vi "商品生成.vi"(11 "天数":i32 min=0 max=31) -> (2 "物品存在索引":i32[](array[numeric]), 3 "市面商品":string[][](array[string]))   [LabVIEW 2011]
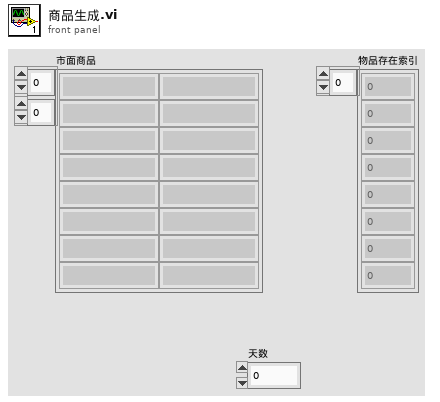
[diagram p1: front panel]
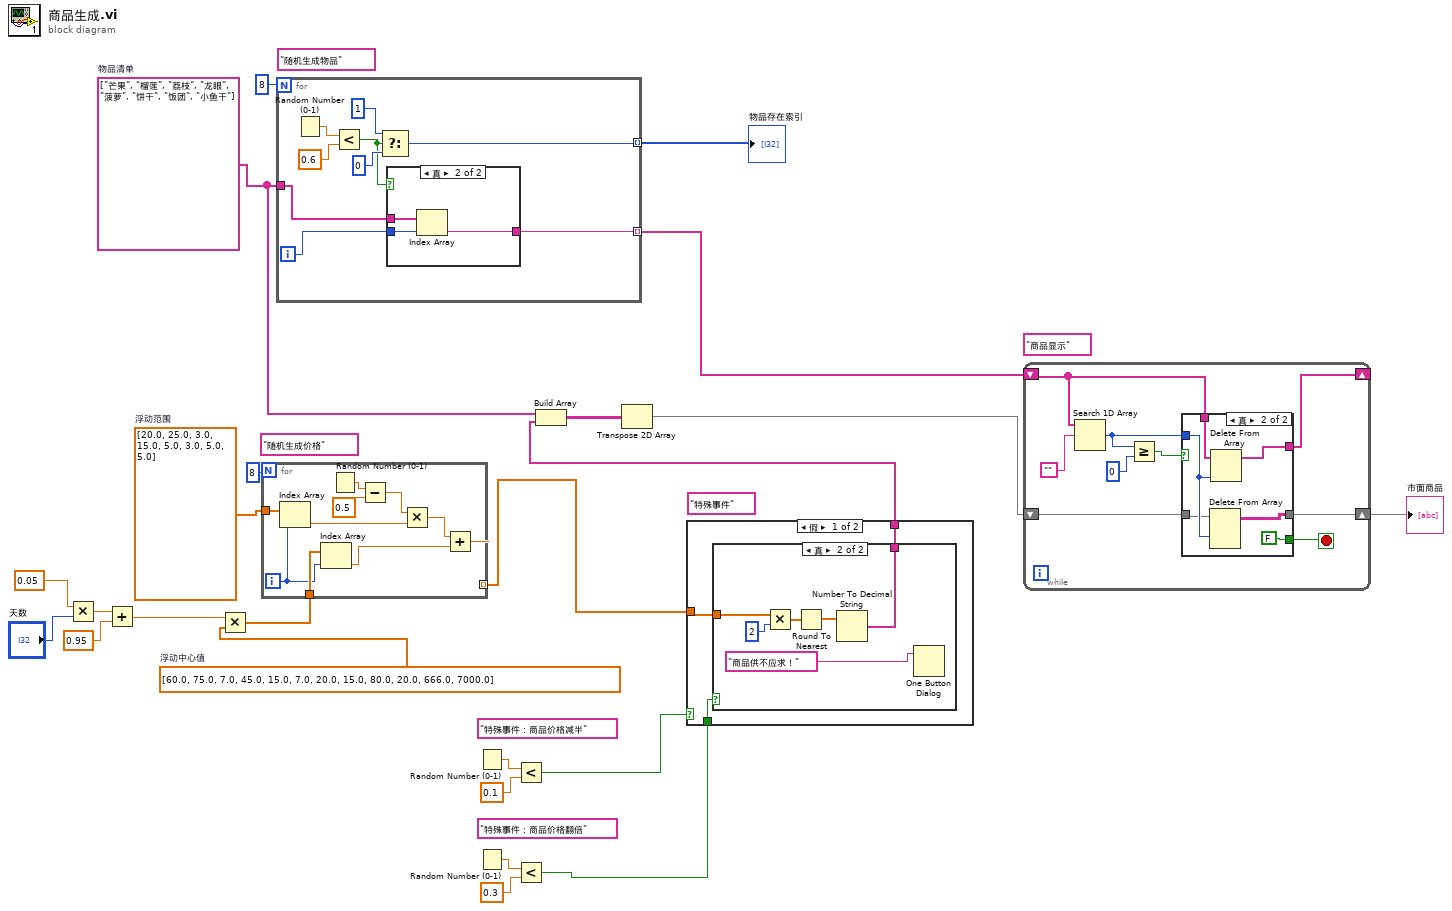
[diagram p0: block diagram]
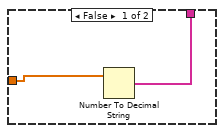
[diagram p2: hidden frame]
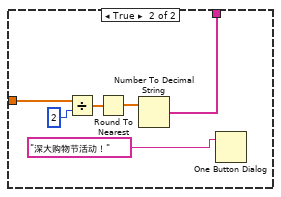
[diagram p3: hidden frame]
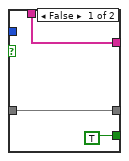
[diagram p4: hidden frame]
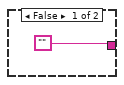
[diagram p5: hidden frame]
diagram:
  (unwired) "商品显示"
  (unwired) "随机生成物品"
  (unwired) "随机生成价格"
  (unwired) "特殊事件"
  (unwired) "特殊事件：商品价格翻倍"
  (unwired) "特殊事件：商品价格减半"
  w19 = string[] ["芒果", "榴莲", "荔枝", "龙眼", "菠萝", "饼干", "饭团", "小鱼干"]  # 物品清单
  w20 = dbl[] [20.0, 25.0, 3.0, 15.0, 5.0, 3.0, 5.0, 5.0]  # 浮动范围
  w3 = dbl[] [60.0, 75.0, 7.0, 45.0, 15.0, 7.0, 20.0, 15.0, 80.0, 20.0, 666.0, 7000.0]  # 浮动中心值
  n1 = Multiply(x=0.05, y="天数") -> (x*y=w4:dbl)
  n2 = Add(x=w4, y=0.95) -> (x+y=w2:dbl)
  n3 = Multiply(x=w2, y=w3) -> (x*y=w1:dbl[])
  n4 = for {
    N: i8 8 -> [_]
    tunnel: [w30] -> w13 mode=indexing
    tunnel: w20 -> [w29]
    tunnel: w1 -> [w27]
    i -> [w25]
    n5 = Index Array(array=w29, index=w25) -> (element=w28:dbl)
    n6 = Index Array(array=w27, index=w25) -> (element=w26:dbl)
    n7 = Random Number (0-1)() -> (number: 0 to 1=w33:dbl)
    n8 = Subtract(x=w33, y=0.5) -> (x-y=w32:dbl)
    n9 = Multiply(x=w32, y=w28) -> (x*y=w31:dbl)
    n10 = Add(x=w31, y=w26) -> (x+y=w30:dbl)
  }
  n11 = for {
    N: i8 8 -> [_]
    tunnel: [w39] -> w18 mode=indexing
    tunnel: w19 -> [w37]
    tunnel: [w35] -> w22 mode=indexing
    i -> [w36]
    n12 = Random Number (0-1)() -> (number: 0 to 1=w43:dbl)
    n13 = Less?(x=w43, y=0.6) -> (x < y?=w38:bool)
    n14 = Select(t=i8 1, s=w38, f=i8 0) -> (s? t:f=w39:i8)
    n15 = case shown="真" w38 {
      tunnel: w37 -> [_ w47]
      tunnel: w36 -> [_ w46]
      tunnel: ["" w45] -> w35
      frame False {
      }
      frame True {
        n16 = Index Array(array=w47, index=w46) -> (element=w45:string)
      }
    }
  }
  "物品存在索引" <- w18
  n17 = Random Number (0-1)() -> (number: 0 to 1=w17:dbl)
  n18 = Random Number (0-1)() -> (number: 0 to 1=w15:dbl)
  n19 = Less?(x=w17, y=0.1) -> (x < y?=w11:bool)
  n20 = Less?(x=w15, y=0.3) -> (x < y?=w10:bool)
  n21 = case shown="假" w11 {
    tunnel: w13 -> [w49 w62]
    tunnel: [w48 w60] -> w12
    tunnel: w10 -> [w50 _]
    frame False {
      n22 = case shown="真" w50 {
        tunnel: w49 -> [w52 w55]
        tunnel: [w51 w54] -> w48
        frame False {
          n23 = Number To Decimal String(number=w52) -> (decimal integer string=w51:string[])  [unwired: 1 in]
        }
        frame True {
          n24 = Multiply(x=w55, y=2) -> (x*y=w57:dbl[])
          n25 = Round To Nearest(number=w57) -> (nearest integer value=w56:dbl[])
          n26 = Number To Decimal String(number=w56) -> (decimal integer string=w54:string[])  [unwired: 1 in]
          n27 = One Button Dialog(message="商品供不应求！") -> ()  [unwired: 1 in, 1 out]
        }
      }
    }
    frame True {
      n28 = Divide(x=w62, y=2) -> (x/y=w63:dbl[])
      n29 = Round To Nearest(number=w63) -> (nearest integer value=w61:dbl[])
      n30 = Number To Decimal String(number=w61) -> (decimal integer string=w60:string[])  [unwired: 1 in]
      n31 = One Button Dialog(message="深大购物节活动！") -> ()  [unwired: 1 in, 1 out]
    }
  }
  n32 = Build Array(w19, w12) -> (w21:string[][])
  n33 = Transpose 2D Array(2D array=w21) -> (transposed array=w9:string[][])
  n34 = while {
    shift-right: [w65] -> _
    shift-left: w22 -> [w70]
    shift-right: [w67] -> w8
    shift-left: w9 -> [w68]
    stop <- w66 stop-if-true
    n35 = Search 1D Array(1D array=w70, element="") -> (index of element=w69:i32)  [unwired: 1 in]
    n36 = Greater Or Equal?(x=w69, y=i8 0) -> (x >= y?=w71:bool)
    n37 = case shown="真" w71 {
      tunnel: w70 -> [w76 w82]
      tunnel: w69 -> [_ w79]
      tunnel: [w76 w81] -> w65
      tunnel: [TRUE FALSE] -> w66
      tunnel: w68 -> [w74 w77]
      tunnel: [w74 w78] -> w67
      frame False {
      }
      frame True {
        n38 = Delete From Array(array=w77, index (row)=w79) -> (array with subset deleted=w78:string[][])  [unwired: 2 in, 1 out]
        n39 = Delete From Array(array=w82, index=w79) -> (array with subset deleted=w81:string[])  [unwired: 1 in, 1 out]
      }
    }
  }
  "市面商品" <- w8
